vi "Get-all-controls-names.vi"() -> (3 "Controls":T1[](array[typedef]))   [LabVIEW 2013, in "CameraVision.lvlib" / "CV-UI.lvclass"]
uses:
  CV-UI.lvclass
  Control-names.ctl
panel:
  in  "Control refs":T1
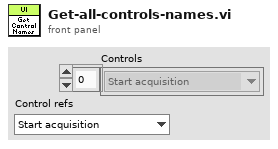
[diagram p1: front panel]
types:
  T1 = typedef "CameraVision.lvlib/CV-UI.lvclass/Control-names.ctl" = enum16{"Start acquisition", "Activate", "Stop acquisition", "Settings type", "Load settings", "Save settings", "Import images", "Camera selector", "Image type selector", "Batch browser", "Image refresh", "Parameter tabs", "Displays", "Processing tabs", "Processing selector", "Map characteristic", "Show info", "Manual trigger"}
  T2 = typedef "CameraVision.lvlib/CV-UI.lvclass/Control-refs.ctl" = enum16{"Start acquisition", "Activate", "Stop acquisition", "Settings type", "Load settings", "Save settings", "Import images", "Camera selector", "Image type selector", "Batch browser", "Image refresh", "Parameter tabs", "Displays", "Processing tabs", "Processing selector", "Map characteristic", "Show info", "Manual trigger"}
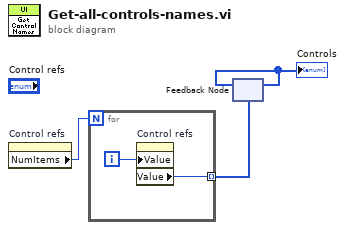
[diagram p0: block diagram]
diagram:
  n1 = property on="Control refs" class="Enum (strict)"() -> ("NumItems"=w2:u32)  [unwired: 2 in, 2 out]
  n2 = for {
    N: w2 -> [_]
    tunnel: [w4] -> w1 mode=indexing
    i -> [w5]
    n3 = property on="Control refs" class="Enum (strict)"("Value"=w5) -> ("Value"=w4:T2)  [unwired: 2 in, 2 out]
  }
  n4 = feedback #1(w1) -> (w3:T2[])
  "Controls" <- w3
  n5 = feedback-in #1(w3) -> ()
